vi "convertMFCOutputBytes.vi"(9 "FullScale":dbl=24576.0, 10 "SCCM":dbl=500.0, 11 "Setpoint":dbl) -> (0 "Byte 1":u8, 3 "Byte 0":u8)   [LabVIEW 2011]
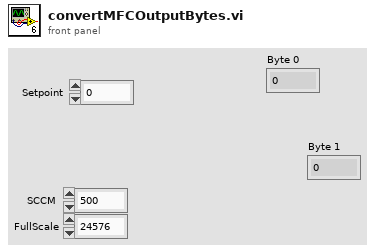
[diagram p1: front panel]
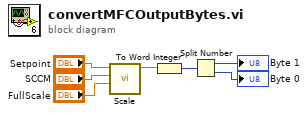
[diagram p0: block diagram]
diagram:
  n1 = call "Scale.vi"("Factor"="FullScale", "FullScale"="SCCM", "Input"="Setpoint") -> ("Output"=w4:dbl)  [unwired: 8 in]
  n2 = To Word Integer(number=w4) -> (16bit integer=w3:i16)
  n3 = Split Number(x=w3) -> (hi(x)=→"Byte 1":u8, lo(x)=→"Byte 0":u8)
